vi "Simple Stream.vi"() -> ()   [LabVIEW 2020]
uses:
  Channel/Channel.lvclass
  Stream/Stream.lvclass
  <vilib>/Utility/config.llb/NI_LVConfig.lvlib
  <vilib>/Utility/config.llb/Read Key (String).vi
panel:
  out "Waveform Chart":dynamicdata(graph)
  out "error out":errorcluster
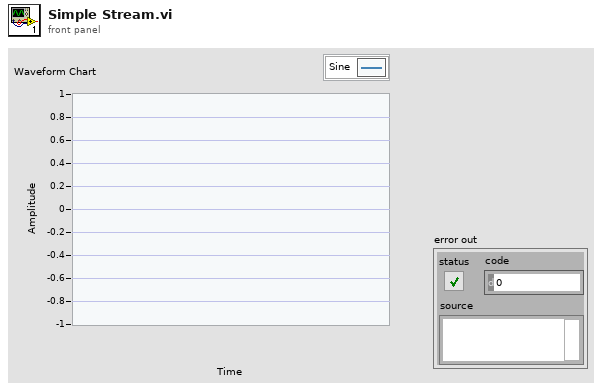
[diagram p1: front panel]
types:
  T1 = typedef "NI_LVConfig.lvlib/Config Data RefNum.ctl" = refnum<k1>
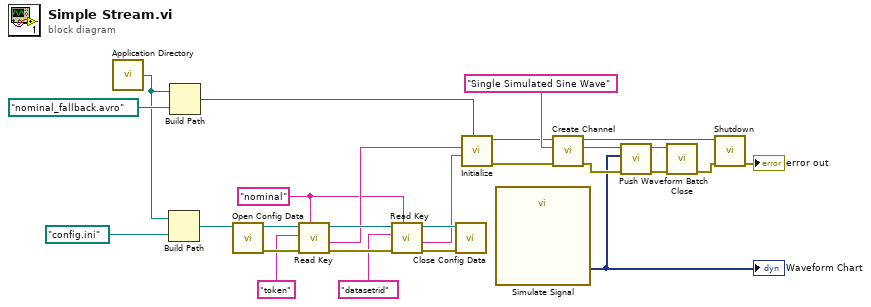
[diagram p0: block diagram]
diagram:
  w1 = "nominal" ("section")
  n1 = call <vilib>:"Application Directory.vi"() -> ("Application Directory"=w18:path)
  n2 = Build Path(base path=w18, name or relative path=path "config.ini") -> (appended path=w12:path)
  n3 = Build Path(base path=w18, name or relative path=path "nominal_fallback.avro") -> (appended path=w19:path)
  n4 = call <vilib>:"Open Config Data.vi"("configuration file path"=w12) -> ("error out"=w6:errorcluster, "refnum"=w11:T1)  [unwired: 8 in, 1 out]
  n5 = call-poly <vilib>:"Read Key.vi"("section"=w1, "error in (no error)"=w6, "key"="token", "refnum"=w11) -> ("error out"=w7:errorcluster, "value"=w2:string, "refnum out"=w10:T1)  [unwired: 4 in, 1 out]
  n6 = call-poly <vilib>:"Read Key.vi"("section"=w1, "error in (no error)"=w7, "key"="datasetrid", "refnum"=w10) -> ("error out"=w8:errorcluster, "value"=w3:string, "refnum out"=w9:T1)  [unwired: 4 in, 1 out]
  n7 = call <vilib>:"Close Config Data.vi"("error in (no error)"=w8, "refnum"=w9) -> ()  [unwired: 8 in, 2 out]
  n8 = call "Initialize.vi"("Fallback File Path"=w19, "Dataset RID"=w3, "Token"=w2) -> ("error out"=w16:errorcluster, "Nominal Streaming out"=w17:refnum<class "Stream.lvclass">)  [unwired: 7 in]
  n9 = call "Simulate Signal"() -> ("Sine"=w14:dynamicdata)  [unwired: 14 in, 1 out]
  "Waveform Chart" <- w14
  n10 = call "Create Channel.vi"("error in (no error)"=w16, "Channel Name"="Single Simulated Sine Wave", "Nominal Streaming in"=w17) -> ("error out"=w24:errorcluster, "Channel"=w25:refnum<class "Channel.lvclass">, "Nominal Streaming out"=w23:refnum<class "Stream.lvclass">)  [unwired: 6 in]
  n11 = call "Push Waveform Batch.vi"("error in (no error)"=w24, "Waveform"=w14, "Channel in"=w25) -> ("error out"=w22:errorcluster, "Channel out"=w26:refnum<class "Channel.lvclass">)  [unwired: 7 in]
  n12 = call "Close.vi"("error in (no error)"=w22, "Channel in"=w26) -> ("error out"=w15:errorcluster)  [unwired: 9 in]
  n13 = call "Shutdown.vi"("error in (no error)"=w15, "Nominal Streaming in"=w23) -> ("error out"=→"error out":errorcluster)  [unwired: 8 in, 1 out]
